vi "Create Error Qs.vi"(8 "error in (no error)":errorcluster) -> (0 "error out":errorcluster, 3 "Error Qs":T1, 5 "Error Publishing Q":refnum<queue>)   [LabVIEW 2016, in "Ballard Arinc-429 Engine.lvlib"]
uses:
  Ballard Arinc-429 Engine.lvlib
  RT Controls/Error Qs.ctl
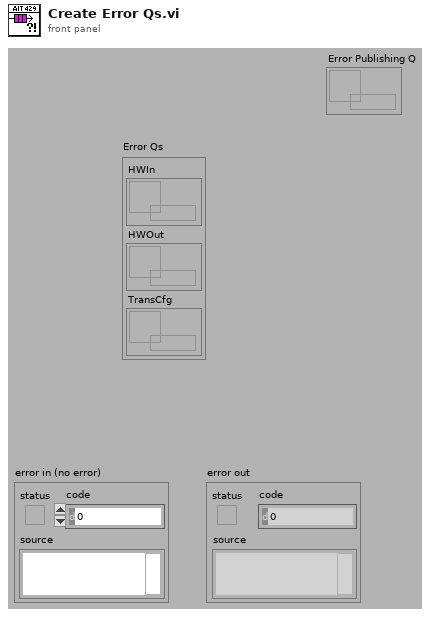
[diagram p1: front panel]
types:
  T1 = typedef "Ballard Arinc-429 Engine.lvlib/Error Qs.ctl" = cluster{"HWIn":refnum<queue>, "HWOut":refnum<queue>, "TransCfg":refnum<queue>}
  T2 = cluster{"[0]":refnum<queue>, "[1]":refnum<queue>, "[2]":refnum<queue>}
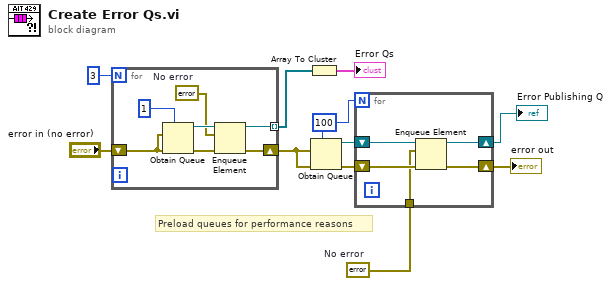
[diagram p0: block diagram]
diagram:
  w5 = errorcluster {"status"=FALSE, "code"=0, "source"=""}  # No error
  w2 = 100 ("max queue size (-1, unlimited)")
  # "Preload queues for performance reasons"
  n1 = for {
    N: 3 -> [_]
    shift-right: [w14] -> w7
    shift-left: "error in (no error)" -> [w18]
    tunnel: [w15] -> w9 mode=indexing
    w12 = errorcluster {"status"=FALSE, "code"=0, "source"=""}  # No error
    n2 = Obtain Queue(max queue size (-1, unlimited)=1, element data type=w18, error in (no error)=w18) -> (queue out=w16:refnum<queue>, error out=w13:errorcluster)  [unwired: 2 in, 1 out]
    n3 = Enqueue Element(queue=w16, element=w12, error in (no error)=w13) -> (queue out=w15:refnum<queue>, error out=w14:errorcluster)  [unwired: 1 in, 1 out]
  }
  n4 = Array To Cluster(array=w9) -> (cluster=→"Error Qs":T2)
  n5 = Obtain Queue(max queue size (-1, unlimited)=w2, element data type=w7, error in (no error)=w7) -> (queue out=w4:refnum<queue>, error out=w6:errorcluster)  [unwired: 2 in, 1 out]
  n6 = for {
    N: w2 -> [_]
    shift-right: [w19] -> w1
    shift-left: w6 -> [w23]
    tunnel: w5 -> [w22]
    shift-right: [w20] -> w3
    shift-left: w4 -> [w21]
    n7 = Enqueue Element(queue=w21, element=w22, error in (no error)=w23) -> (queue out=w20:refnum<queue>, error out=w19:errorcluster)  [unwired: 1 in, 1 out]
  }
  "error out" <- w1
  "Error Publishing Q" <- w3
